vi "Mixer subVI.vi"(10 "Reference in":waveform(dbl), 11 "Signal in":waveform(dbl)) -> (3 "Signal*Reference out":waveform(dbl))   [LabVIEW 2019, in "DSP.lvclass"]
uses:
  DSP.lvclass
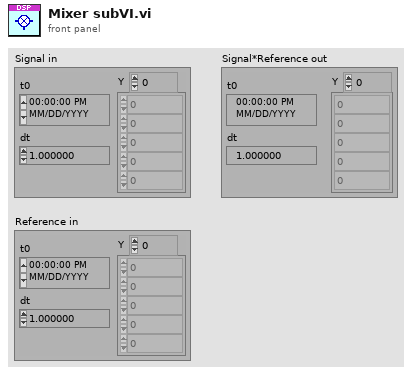
[diagram p1: front panel]
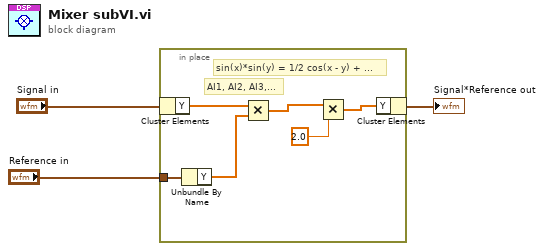
[diagram p0: block diagram]
diagram:
  n1 = in-place {
    in-place-border: "Reference in" -> [w8]
    # "sin(x)*sin(y) = 1/2 cos(x - y) + ..."
    # "AI1, AI2, AI3,..."
    n2 = in-place-cluster #1("Signal in") -> ("Y"=w9:dbl[])
    n3 = Unbundle By Name(w8) -> ("Y"=w7:dbl[])
    n4 = Multiply(x=w9, y=w7) -> (x*y=w6:dbl[])
    n5 = Multiply(x=w6, y=2.0) -> (x*y=w5:dbl[])
    n6 = in-place-cluster #1("Y"=w5) -> (→"Signal*Reference out":waveform(dbl))
  }
